vi "get postion.vi"(10 "Array":dbl[](array[numeric]), 11 "get and go Position in":T1) -> (3 "get and go Position out":T1)   [LabVIEW 2016]
panel:
  out "output array":dbl[][](array[numeric])
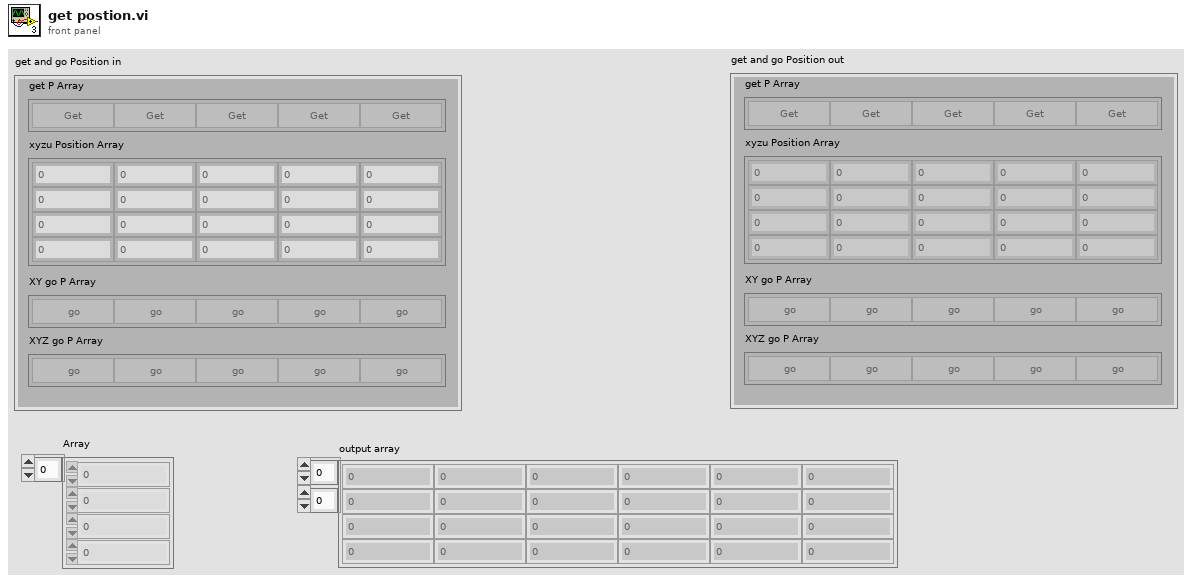
[diagram p1: front panel]
types:
  T1 = cluster{"get P Array":bool[], "XY go P Array":bool[], "xyzu Position Array":dbl[][], "XYZ go P Array":bool[]}
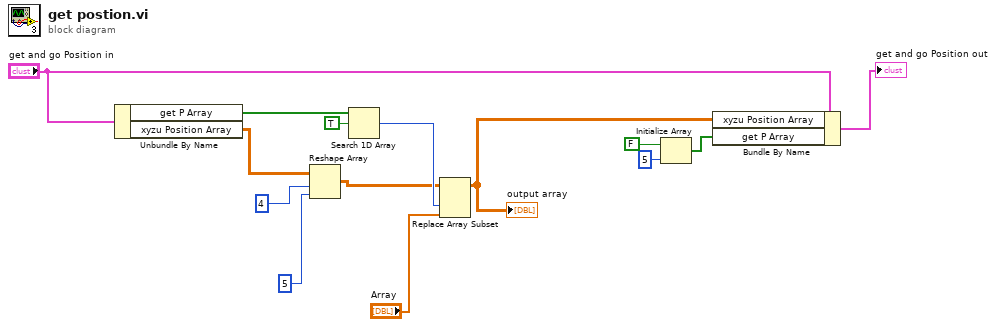
[diagram p0: block diagram]
diagram:
  n1 = Unbundle By Name("get and go Position in") -> ("get P Array"=w14:bool[], "xyzu Position Array"=w6:dbl[][])
  n2 = Reshape Array "Reshape Array"(w6, 4 ("dimension size"), 5 ("dimension size")) -> (w7:dbl[][])
  n3 = Search 1D Array(1D array=w14, element=TRUE) -> (index of element=w12:i32)  [unwired: 1 in]
  n4 = Replace Array Subset "Replace Array Subset"(array=w7, new element="Array", index (col)=w12) -> (w8:dbl[][])  [unwired: 1 in]
  "output array" <- w8
  n5 = Initialize Array(FALSE, 5 ("dimension size")) -> (w1:bool[])
  n6 = Bundle By Name(cluster="get and go Position in", "xyzu Position Array"=w8, "get P Array"=w1) -> (→"get and go Position out":T1)
